vi "Delete Uint64Array DVR.vi"(8 "error in (no error)":errorcluster, 11 "Uint64Array DVR in":refnum<data-value>) -> (0 "error out":errorcluster, 3 "Uint64Array out":refnum<class "Uint64Array.lvclass">)   [LabVIEW 2012, in "MDSplus.lvlib" / "Uint64Array.lvclass"]
uses:
  <vilib>/MDSplus/Classes/Data_Class/Array_Class/Uint64Array_Class/Uint64Array.lvclass
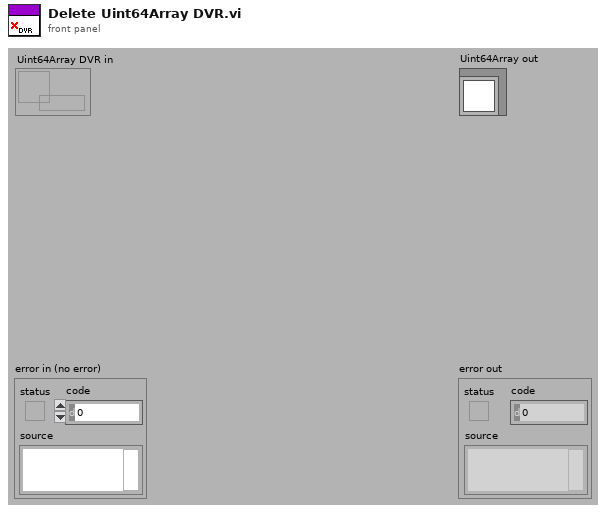
[diagram p1: front panel]
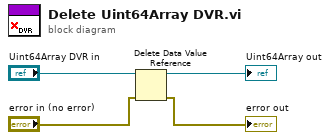
[diagram p0: block diagram]
diagram:
  n1 = Delete Data Value Reference(data value reference="Uint64Array DVR in", error in="error in (no error)") -> (data value=→"Uint64Array out":refnum<class "Uint64Array.lvclass">, error out=→"error out":errorcluster)
